vi "acquireTempWF.vi"() -> ()   [LabVIEW 2020]
uses:
  <instrlib>/niScope/Acquire/Fetch/niScope Multi Fetch Binary 16.vi
panel:
  out "Ch3 Graph":dbl[](graph)
  out "Ch2 Graph":dbl[](graph)
  out "Ch1 Graph":dbl[](graph)
  in  "Acquire Button":bool
  out "Error Out":errorcluster
  in  "Bias":dbl format="%.2f"
  out "Record Backlog":i32
  out "Dig2 Records Done":i32
  out "Aquisition loop timing":u32
  in  "Error In":errorcluster
  in  "niTClk sessions":refnum<k20>[](array[refnum])
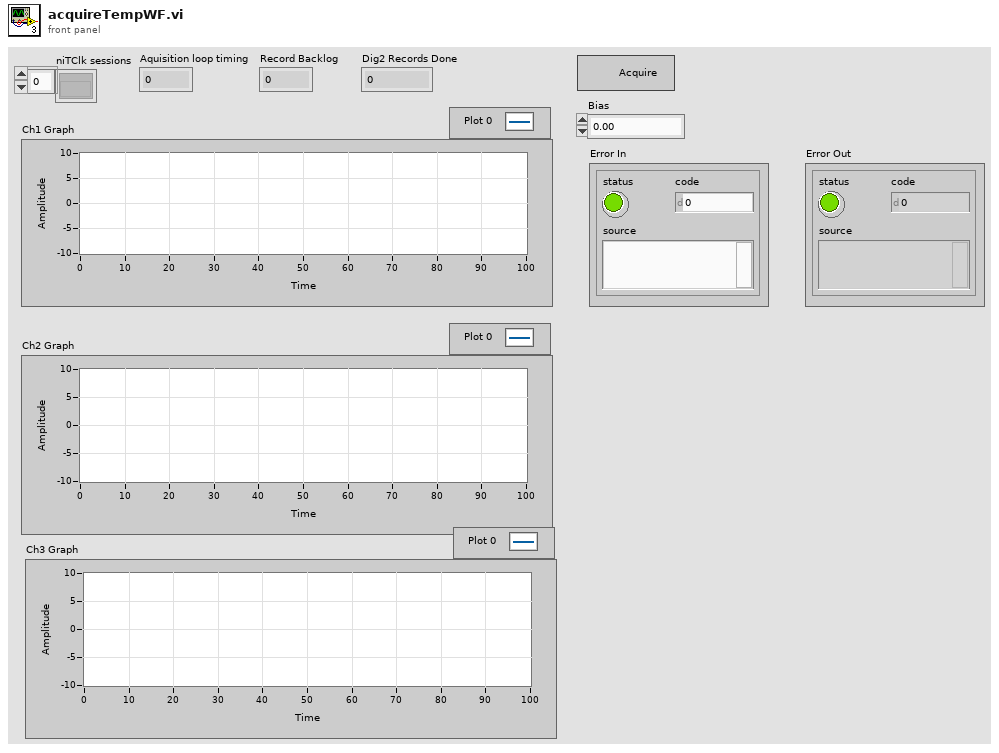
[diagram p1: front panel]
types:
  T1 = typedef "FLImDAQ.ctl" = cluster{"Digitizer 1":refnum<k15>, "Digitizer 2":refnum<k15>, "Channel":enum16{"Channel 0", "Channel 1", "Channel 0&1"}, "trigger source":T2, "trigger level":dbl, "trigger delay":dbl, "min sample rate":dbl, "min record length":i32, "vertical range":dbl, "vertical offset":dbl, "Waveform to Avg":i16}
  T2 = typedef "niScope trigger source.ctl" = string
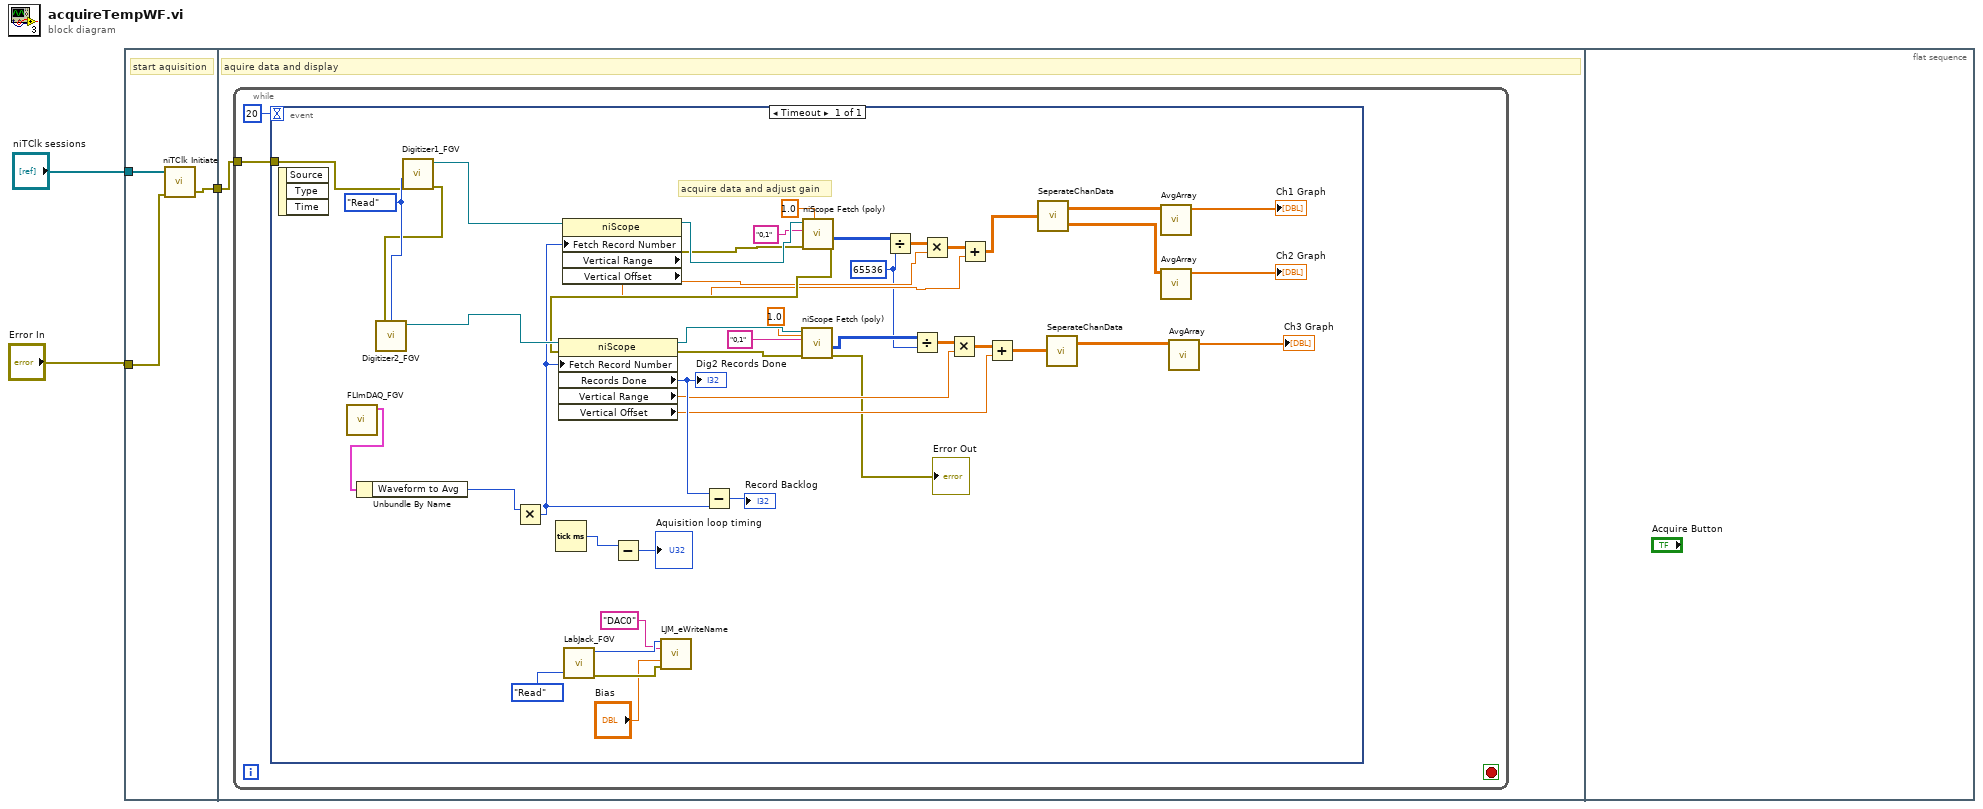
[diagram p0: block diagram]
diagram:
  n1 = flat-sequence {
    tunnel: "niTClk sessions" -> [w6]
    tunnel: "Error In" -> [w5]
    tunnel: [w4] -> w1
    tunnel: w1 -> [w7]
    frame #0 {
      # "start aquisition"
      n2 = call <instrlib>:"niTClk Initiate.vi"("error in (no error)"=w5, "sessions"=w6) -> ("error out"=w4:errorcluster)  [unwired: 8 in, 1 out]
    }
    frame #1 {
      # "aquire data and display"
      n3 = while {
        tunnel: w7 -> [w8]
        stop <- _ stop-if-true
        n4 = event shown="[0] Timeout" {
          selector: _ -> [_]
          dyn-events: _ -> [_]
          timeout: 20 -> [_]
          tunnel: w8 -> [w50]
          event Timeout {
            w28 = 65536
            w56 = enum16{"Write", "Read"}."Read" ("Operation")
            # "acquire data and adjust gain"
            n5 = event-data() -> ()  [unwired: 1 in, 3 out]
            n6 = call "FLImDAQ_FGV.vi"() -> ("Read data"=w52:T1)  [unwired: 10 in, 1 out]
            n7 = Unbundle By Name(w52) -> ("Waveform to Avg"=w51:i16)
            n8 = call "Digitizer1_FGV.vi"("error in (no error)"=w50, "Operation (Read)"=w56) -> ("error out"=w55:errorcluster, "Read data"=w54:refnum<k15>)  [unwired: 8 in]
            n9 = call "Digitizer2_FGV.vi"("error in (no error)"=w55, "Operation (Read)"=w56) -> ("Read data"=w53:refnum<k15>)  [unwired: 8 in, 1 out]
            n10 = Multiply(x=w51) -> (x*y=w39:i16)  [unwired: 1 in]
            n11 = Tick Count (ms)() -> (millisecond timer value=w27:u32)
            n12 = property class="niScope"(reference=w54, "Fetch Record Number"=w39) -> (reference out=w49:refnum<k15>, error out=w48:errorcluster, "Vertical Range"=w37:dbl, "Vertical Offset"=w35:dbl)  [unwired: 1 in]
            n13 = call "LabJack_FGV.vi"("Operation(Read)"=enum16{"Write", "Read"}."Read" ("Operation")) -> ("error out"=w21:errorcluster, "Read data"=w22:i32)  [unwired: 9 in]
            n14 = Subtract(x=w27) -> (y=w26:u32, x-y=→"Aquisition loop timing":u32)
            n15 = call "LJM_eWriteName.vi"("Handle In"=w22, "Name"="DAC0", "Value"="Bias", "error in"=w21) -> ()  [unwired: 10 in, 2 out]
            n16 = call-poly <instrlib>:"niScope Fetch (poly).vi"("timeout"=1.0, "error in"=w48, "channels"="0,1", "instrument handle"=w49) -> ("error out"=w40:errorcluster, "wfm"=w24:i16[][])  [unwired: 4 in, 2 out]
            n17 = property class="niScope"(reference=w53, error in=w40, "Fetch Record Number"=w39) -> (reference out=w44:refnum<k15>, error out=w41:errorcluster, "Records Done"=w34:i32, "Vertical Range"=w30:dbl, "Vertical Offset"=w29:dbl)
            "Dig2 Records Done" <- w34
            n18 = Subtract(x=w34, y=w39) -> (x-y=→"Record Backlog":i32)
            n19 = call-poly <instrlib>:"niScope Fetch (poly).vi"("timeout"=1.0, "error in"=w41, "channels"="0,1", "instrument handle"=w44) -> ("error out"=→"Error Out":errorcluster, "wfm"=w31:i16[][])  [unwired: 4 in, 2 out]
            n20 = Divide(x=w24, y=w28) -> (x/y=w38:dbl[][])
            n21 = Divide(x=w31, y=w28) -> (x/y=w33:dbl[][])
            n22 = Multiply(x=w38, y=w37) -> (x*y=w36:dbl[][])
            n23 = Multiply(x=w33, y=w30) -> (x*y=w32:dbl[][])
            n24 = Add(x=w36, y=w35) -> (x+y=w15:dbl[][])
            n25 = Add(x=w32, y=w29) -> (x+y=w13:dbl[][])
            n26 = call "SeperateChanData.vi"("Input (Ch1&2)"=w15) -> ("Ch1"=w17:dbl[][], "Ch2"=w16:dbl[][])
            n27 = call "SeperateChanData.vi"("Input (Ch1&2)"=w13) -> ("Ch1"=w14:dbl[][])  [unwired: 1 out]
            n28 = call "AvgArray.vi"("2D array in"=w17) -> ("1D Avg out"=→"Ch1 Graph":dbl[])  [unwired: 10 in]
            n29 = call "AvgArray.vi"("2D array in"=w16) -> ("1D Avg out"=→"Ch2 Graph":dbl[])  [unwired: 10 in]
            n30 = call "AvgArray.vi"("2D array in"=w14) -> ("1D Avg out"=→"Ch3 Graph":dbl[])  [unwired: 10 in]
          }
        }
      }
    }
    frame #2 {
    }
  }
